vi "Check_Beam_Powers.vi"(3 "Mode":T5, 5 "Traverse line In":T2 {"Carrier_2 Q (l/min)" format="%#.2f"; "Row Duration (mins)" format="%#.1f"; "Row No" min=0; "Trace Gas Concentration (%)" min=0.0 format="%#_4f"; "Carrier_1 Q (l/min)" format="%#.4f"; "Start X" format="%#.2f"; "Start Y" format="%#.2f"; "Start Z" format="%#.2f"; "End X" format="%#.2f"; "End Y" format="%#.2f"; "End Z" format="%#.2f"; "Tunnel Speed" format="%#.2f"; "Averaging time (mins)" min=0.0 format="%#.2f"}) -> (0 "Error Message":string, 1 "Status":T1, 2 "Traverse line Out":T2 {"Carrier_2 Q (l/min)" format="%#.2f"; "Row Duration (mins)" format="%#.1f"; "Row No" min=0; "Trace Gas Concentration (%)" min=0.0 format="%#_4f"; "Carrier_1 Q (l/min)" format="%#.4f"; "Start X" format="%#.2f"; "Start Y" format="%#.2f"; "Start Z" format="%#.2f"; "End X" format="%#.2f"; "End Y" format="%#.2f"; "End Z" format="%#.2f"; "Tunnel Speed" format="%#.2f"; "Averaging time (mins)" min=0.0 format="%#.2f"})   [LabVIEW 2021]
uses:
  Gen Trav/Traverse_cluster.ctl
  Gen Trav/Spacing.ctl
  Controls/Multi_run_mode.ctl
  Controls/User_Specific_mode.ctl
  Gen Trav/Multi_Run_Status.ctl
  Gen Trav/Trav_mode.ctl
  Controls/Tunnel_Coordinates.ctl
panel:
  out "Min  Acceptable Power":dbl[](array[numeric]) format="%.3f"
  out "Initially Mirror Up?":bool
  out "Mirror Installed":string
  out "Waveform Graph":dbl[][](graph)
  out "beams to check":i32
  out "Beam Data":sgl[][](array[numeric])
  out "Light Power (mW)":dbl=8.10606551e-08 format="%#.3f"
  in  "stop":bool
  out "Powers":dbl[](array[numeric]) format="%.3f"
  out "Beam Index":i32
  # "X                      Y                   Z"
  # "X           Y          Z"
  # "Start"
  # "End"
  # "X           Y          Z"
  # "Start"
  # "End"
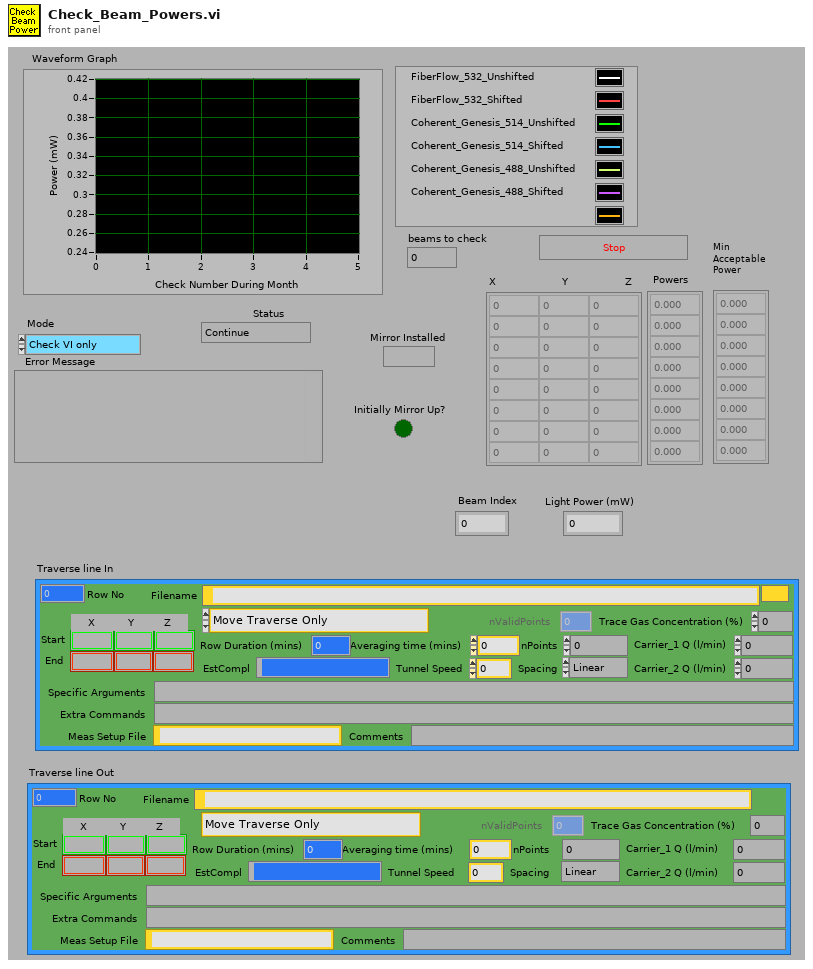
[diagram p1: front panel]
types:
  T1 = typedef "Multi_Run_Status.ctl" = enum16{"Continue", "Continue with Error", "Jump to Next Point", "Jump to Next Row", "Jump To Fall Back", "Terminate Run"}
  T2 = typedef "Traverse_cluster.ctl" = cluster{"Start X":sgl, "Start Y":sgl, "Start Z":sgl, "End X":sgl, "End Y":sgl, "End Z":sgl, "nPoints":i32, "Spacing":T3, "Filename":path, "Tunnel Speed":dbl, "Averaging time (mins)":dbl, "Extra Commands":string, "Carrier_1 Q (l/min)":dbl, "Carrier_2 Q (l/min)":dbl, "Trace Gas Concentration (%)":dbl, "Specific Arguments":string, "Comments":string, "Row No":i32, "Row Type Selector":T4, "EstCompl":string, "Row Duration (mins)":dbl, "nValidPoints":i32, "Meas Setup File":string}
  T3 = typedef "Spacing.ctl" = enum16{"Linear", "Log", "Gauss", "Specified", "N/A"}
  T4 = typedef "Multi_run_mode.ctl" = enum16{"Move Traverse Only", "Set Tunnel Speed Only", "Set Source Only", "Set Measurement Conditions", "Single Measurement", "Vertical Profile", "Lateral Profile", "Longitudinal Profile", "Multi-Axis Profile", "Explore Volume", "Auto Calibrate", "Meas Fast FID Bkgnd", "Check Beam Power", "Scanning Valve Measurement", "Run VI Named:", "Set ADAM Ch", "Wait (minutes)", "Send Message", "Synchronize With:", "Fall Back to this Row", "Turn Off Row Repeating", "Traverse 3D Volume", "Blank Row", "Jump to Fall Back Row"}
  T5 = typedef "User_Specific_mode.ctl" = enum16{"Check VI only", "Run VI"}
  T6 = cluster{"Position":dbl[], "Traverse Name":string}[][]
  T7 = typedef "Tunnel_Coordinates.ctl" = enum16{"Work in Tunnel Coordinates", "Work in Model Coordinates"}
  T8 = typedef "Trav_mode.ctl" = enum16{"Move traverse", "Read traverse position", "Teach Position"}
  T9 = cluster{"Position":dbl[], "Traverse Name":string}[]
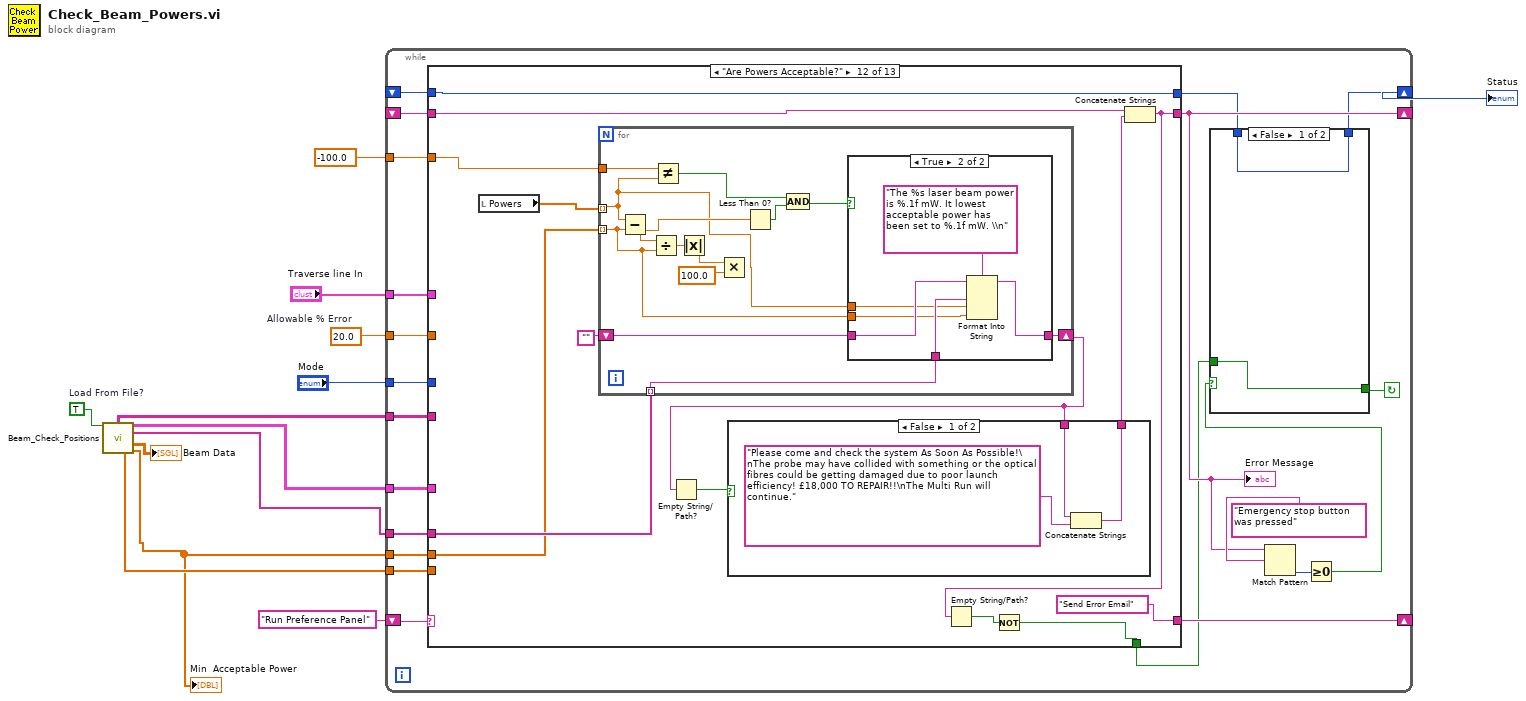
[diagram p0: block diagram]
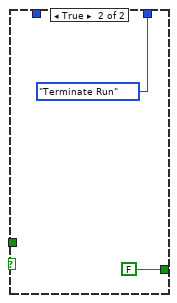
[diagram p2: hidden frame]
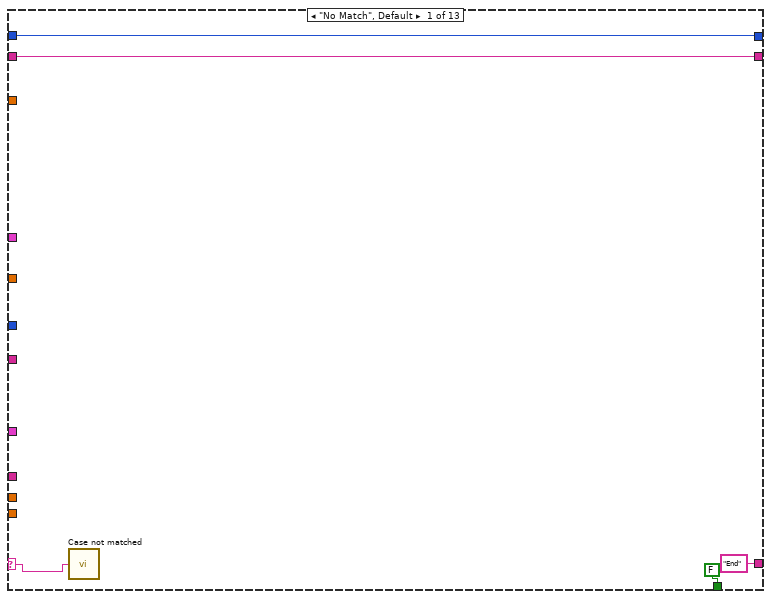
[diagram p3: hidden frame]
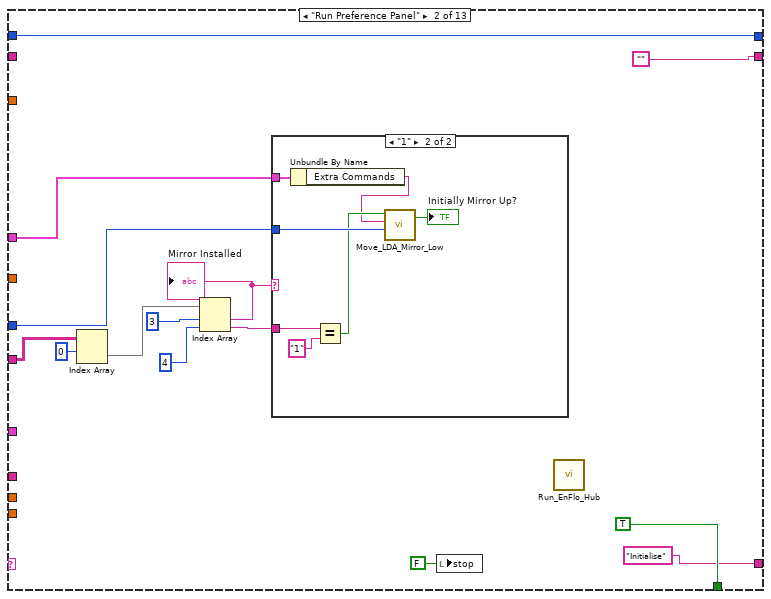
[diagram p4: hidden frame]
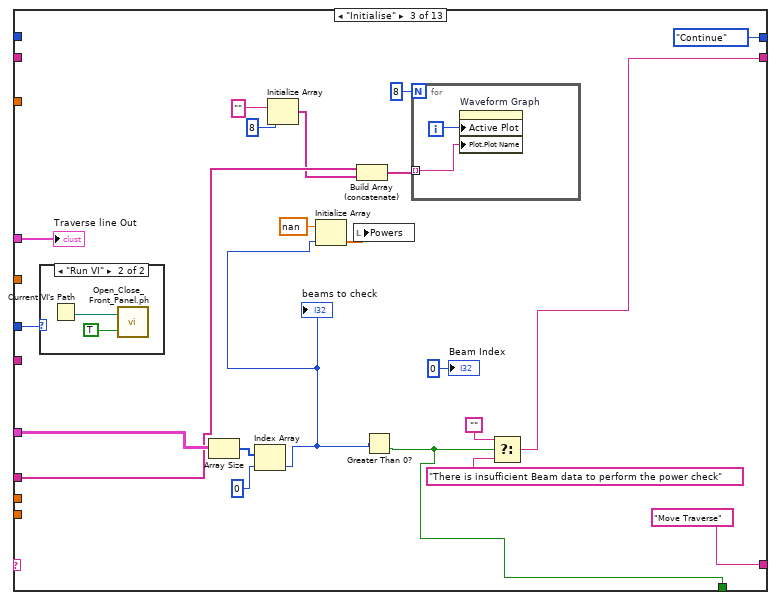
[diagram p6: hidden frame]
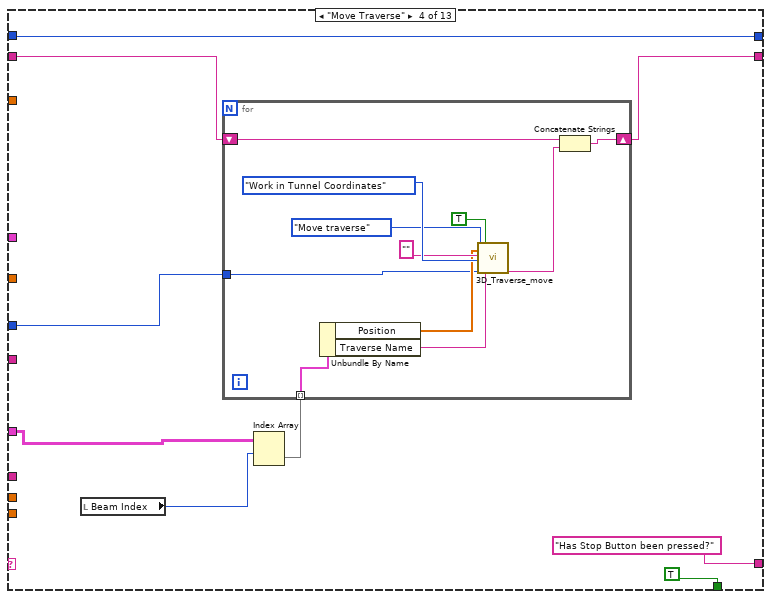
[diagram p8: hidden frame]
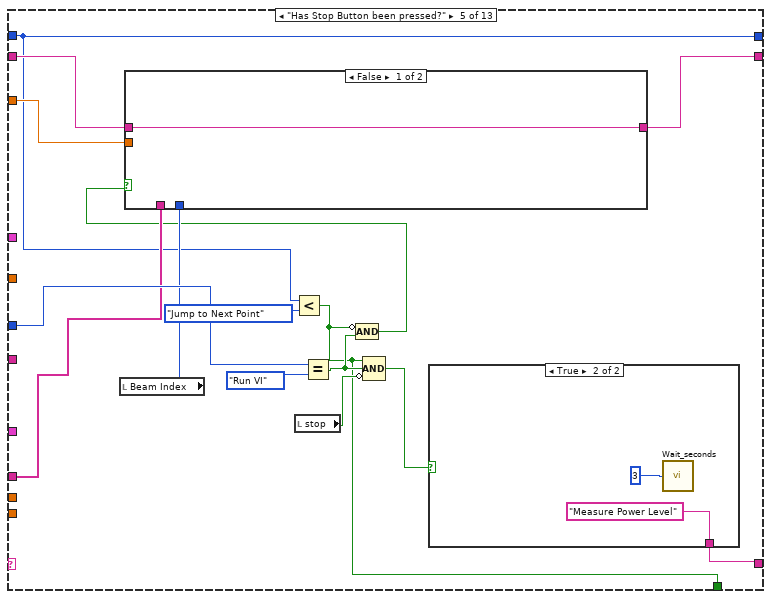
[diagram p9: hidden frame]
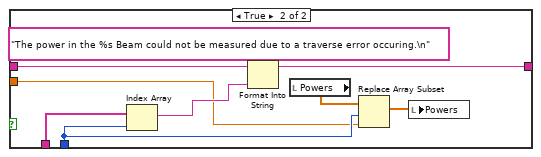
[diagram p10: hidden frame]
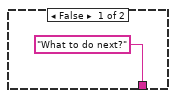
[diagram p11: hidden frame]
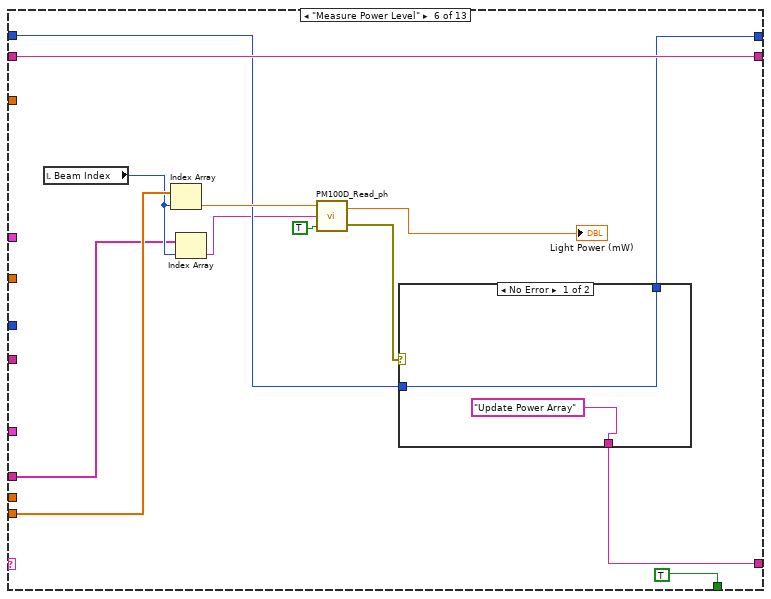
[diagram p12: hidden frame]
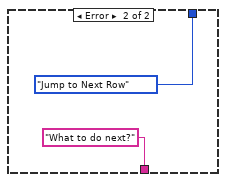
[diagram p13: hidden frame]
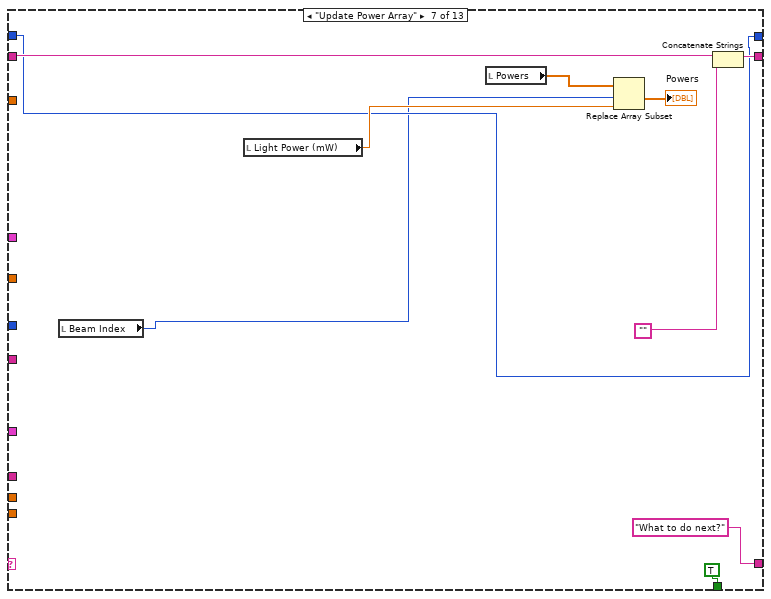
[diagram p14: hidden frame]
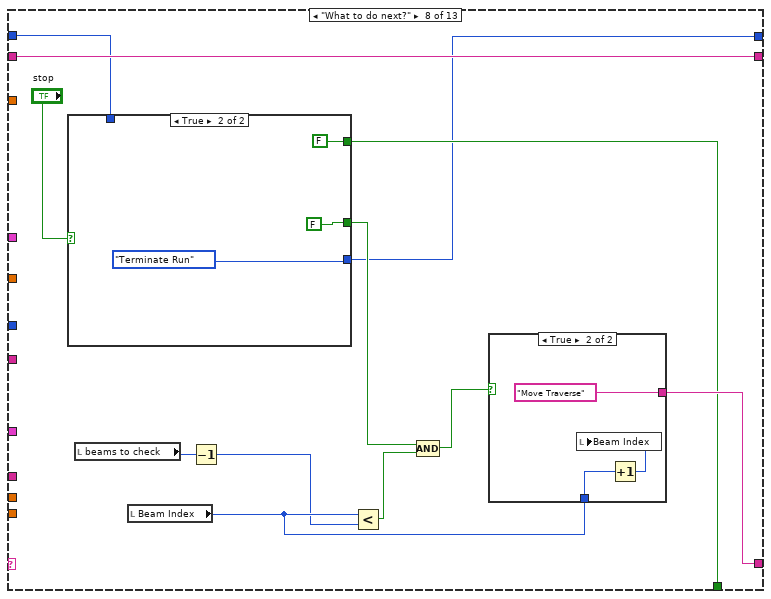
[diagram p15: hidden frame]
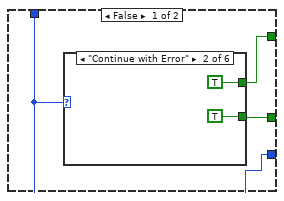
[diagram p16: hidden frame]
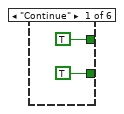
[diagram p17: hidden frame]
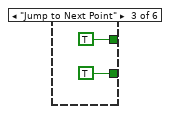
[diagram p18: hidden frame]
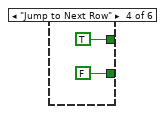
[diagram p19: hidden frame]
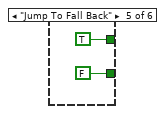
[diagram p20: hidden frame]
diagram:
  w7 = TRUE  # Load From File?
  w11 = 20.0  # Allowable % Error
  n1 = call "Beam_Check_Positions.vi"("Load From File?"=w7) -> ("More Info"=w2:string[][], "Beam Info"=w5:T6, "Beam Names"=w4:string[], "Primary Beam Positions"=→"Beam Data":dbl[][], "Wavelength (nm)"=w3:dbl[], "Power (mW)"=w1:dbl[])  [unwired: 6 in, 3 out]
  "Min  Acceptable Power" <- w1
  n2 = while {
    tunnel: -100.0 ("Element Data") -> [w27]
    tunnel: w11 -> [w29]
    shift-left: _ -> [w30]
    shift-right: [w19] -> _
    tunnel: w4 -> [w32]
    tunnel: "Traverse line In" -> [w33]
    tunnel: "Mode" -> [w34]
    shift-left: "Run Preference Panel" -> [w28]
    shift-right: [w31] -> _
    shift-right: [w15] -> w8
    shift-left: _ -> [w26]
    tunnel: w1 -> [w25]
    tunnel: w5 -> [w24]
    tunnel: w3 -> [w23]
    tunnel: w2 -> [w22]
    stop <- w17 continue-if-true
    n3 = case shown="\"Are Powers Acceptable?\"" w28 {
      selector: w28 -> [w39 _ _ _ _ _ _ _ _ _ _ _ _]
      tunnel: w33 -> [_ w44 w85 _ _ _ _ _ _ w207 _ _ _]
      tunnel: w34 -> [_ w47 w84 w90 w122 _ _ _ w203 w205 _ _ _]
      tunnel: w32 -> [_ _ w67 _ w120 w139 _ _ _ w210 _ w261 _]
      tunnel: [FALSE ("Update Datum Powers?") TRUE ("Update Datum Powers?") w78 TRUE w111 TRUE TRUE w169 w199 TRUE ("Update Datum Powers?") w229 w250 FALSE ("Update Datum Powers?")] -> w16
      tunnel: ["End" "Initialise" "Move Traverse" "Has Stop Button been pressed?" w121 w141 "What to do next?" w171 "Log Beam Power Readings" "Is Laser on Full Power?" ("f") "Are Powers Acceptable?" ("f") "Send Error Email" "End"] -> w31
      tunnel: w30 -> [w41 _ _ w94 w118 w149 w161 w173 w202 w213 w226 w259 w291]
      tunnel: [w41 "" w79 w93 w119 w149 w160 w173 w202 w213 w226 w249 ""] -> w19
      tunnel: w29 -> [_ _ _ _ _ _ _ _ _ _ _ _ _]
      tunnel: w27 -> [_ _ _ _ w117 _ _ _ _ _ _ w257 _]
      tunnel: [w40 w56 Multi_Run_Status."Continue" ("Status") w92 w110 w143 w156 w167 w201 w214 w227 w256 w287] -> w14
      tunnel: w26 -> [w40 w56 _ w92 w110 w142 w156 w168 w201 w214 w227 w256 w287]
      tunnel: w25 -> [_ _ _ _ _ _ _ _ _ _ _ w252 _]
      tunnel: w24 -> [_ _ w74 w91 _ _ _ _ _ _ _ _ _]
      tunnel: w23 -> [_ _ _ _ _ w147 _ _ _ _ _ _ _]
      tunnel: w22 -> [_ w52 _ _ _ _ _ _ _ _ w233 _ _]
      frame "No Match", Default {
        n4 = call "Case not matched.vi"("Case Name not Matched"=w39) -> ()
      }
      frame "Run Preference Panel" {
        n5 = Index Array(array=w52, index (row)=0) -> (element=w50:string[])  [unwired: 1 in]
        n6 = Index Array(array=w50, index #1=3 ("index"), index #2=4 ("index")) -> (element #1=w46:string, element #2=w45:string)
        "Mirror Installed" <- w46
        n7 = case shown="\"1\"" w46 {
          tunnel: w47 -> [_ w64]
          tunnel: w45 -> [_ w63]
          tunnel: w44 -> [_ w60]
          frame Default {
          }
          frame "1" {
            n8 = Unbundle By Name(w60) -> ("Extra Commands"=w59:string)
            n9 = Equal?(x=w63, y="1") -> (x = y?=w61:bool)
            n10 = call "Move_LDA_Mirror_Low.vi"("Mode"=w64, "Extra Commands"=w59, "Mirror Up?"=w61) -> ("Initially Mirror Up?"=→"Initially Mirror Up?":bool)  [unwired: 1 in, 1 out]
          }
        }
        n11 = local write "stop"(FALSE ("stop")) -> ()
        n12 = call "Run_EnFlo_Hub.vi"() -> ()  [unwired: 1 in, 7 out]
      }
      frame "Initialise" {
        n13 = case shown="\"Run VI\"" w84 {
          frame "Check VI only" {
          }
          frame "Run VI" {
            n14 = Current VI's Path() -> (path=w88:path)
            n15 = call "Open_Close_Front_Panel.ph.vi"("openWindow (T)"=TRUE ("Front Panel Window:Open"), "VI path"=w88) -> ()  [unwired: 2 out]
          }
        }
        n16 = Array Size(array=w74) -> (size(s)=w77:i32[])
        n17 = Index Array(array=w77, index=0) -> (element=w71:i32)
        "beams to check" <- w71
        n18 = Initialize Array("", 8 ("dimension size")) -> (w66:string[])
        n19 = Initialize Array(nan ("Numeric"), w71) -> (w73:dbl[])
        n20 = local write "Powers"(w73) -> ()
        n21 = Build Array (concatenate)(w67, w66) -> (w65:string[])
        n22 = Greater Than 0?(x=w71) -> (x > 0?=w78:bool)
        n23 = for {
          N: 8 -> [_]
          tunnel: w65 -> [w87] mode=indexing
          i -> [w86]
          n24 = property on="Waveform Graph" class="WFGraph (strict)"("Active Plot"=w86, "Plot.Plot Name"=w87) -> ()  [unwired: 2 in, 2 out]
        }
        n25 = Select(t="", s=w78, f="There is insufficient Beam data to perform the power check") -> (s? t:f=w79:string)
        "Beam Index" <- 0 ("Numeric")
        "Traverse line Out" <- w85
      }
      frame "Move Traverse" {
        n26 = local read "Beam Index"() -> (w96:i32)
        n27 = Index Array(array=w91, index (row)=w96) -> (element=w95:T9)  [unwired: 1 in]
        n28 = for {
          tunnel: w95 -> [w105] mode=indexing
          shift-right: [w102] -> w93
          shift-left: w94 -> [w101]
          tunnel: w90 -> [w99]
          n29 = Unbundle By Name(w105) -> ("Position"=w104:dbl[], "Traverse Name"=w103:string)
          n30 = call "3D_Traverse_move.vi"("Mode"=Trav_mode."Move traverse", "Position"=w104, "Extra command String"="", "Work in Tunnel Coordinates"=Tunnel_Coordinates."Work in Tunnel Coordinates", "Simulate/Run"=w99, "Route Checking?"=TRUE, "Traverse name"=w103) -> ("Error String"=w100:string)  [unwired: 9 in, 3 out]
          n31 = Concatenate Strings(w101, w100) -> (w102:string)
        }
      }
      frame "Has Stop Button been pressed?" {
        n32 = local read "Beam Index"() -> (w116:i32)
        n33 = Less?(x=w110, y=Multi_Run_Status."Jump to Next Point" ("Status")) -> (x < y?=w111:bool)
        n34 = local read "stop"() -> (w115:bool)
        n35 = Equal?(x=w122, y=User_Specific_mode."Run VI" ("Mode")) -> (x = y?=w113:bool)
        n36 = Compound Arithmetic op=AND(invert w111, w113) -> (w112:bool)
        n37 = case shown="False" w112 {
          tunnel: w116 -> [_ w127]
          tunnel: w120 -> [_ w134]
          tunnel: w118 -> [w125 w131]
          tunnel: [w125 w130] -> w119
          tunnel: w117 -> [_ w126]
          frame False {
          }
          frame True {
            n38 = Index Array(array=w134, index=w127) -> (element=w133:string)
            n39 = Format Into String(format string="The power in the %s Beam could not be measured due to a traverse error occuring.\n" ("Format String"), initial string=w131, w133) -> (resulting string=w130:string)  [unwired: 1 in, 1 out]
            n40 = local read "Powers"() -> (w129:dbl[])
            n41 = Replace Array Subset(array=w129, new element=w126, index=w127) -> (w128:dbl[])
            n42 = local write "Powers"(w128) -> ()
          }
        }
        n43 = Compound Arithmetic op=AND(w111, w113, invert w115) -> (w114:bool)
        n44 = case shown="True" w114 {
          tunnel: ["What to do next?" "Measure Power Level"] -> w121
          frame False {
          }
          frame True {
            n45 = call "Wait_seconds.vi"("Seconds to wait"=u32 3) -> ()
          }
        }
      }
      frame "Measure Power Level" {
        n46 = local read "Beam Index"() -> (w140:i32)
        n47 = Index Array(array=w147, index=w140) -> (element=w146:dbl)
        n48 = Index Array(array=w139, index=w140) -> (element=w138:string)
        n49 = call "PM100D_Read_ph.vi"("stop"=TRUE, "Beam Name"=w138, "Wavelength (0.0)"=w146) -> ("error out"=w144:errorcluster, "Average Power (mW)"=→"Light Power (mW)":dbl)
        n50 = case shown="No Error" w144 {
          tunnel: [w152 Multi_Run_Status."Jump to Next Row" ("Status")] -> w143
          tunnel: w142 -> [w152 _]
          tunnel: ["Update Power Array" "What to do next?"] -> w141
          frame No Error {
          }
          frame Error {
          }
        }
      }
      frame "Update Power Array" {
        n51 = local read "Beam Index"() -> (w155:i32)
        n52 = local read "Light Power (mW)"() -> (w157:dbl)
        n53 = local read "Powers"() -> (w163:dbl[])
        n54 = Replace Array Subset(array=w163, new element=w157, index=w155) -> (→"Powers":dbl[])
        n55 = Concatenate Strings(w161, "") -> (w160:string)
      }
      frame "What to do next?" {
        n56 = case shown="True" "stop" {
          tunnel: [w179 FALSE] -> w170
          tunnel: [w178 FALSE] -> w169
          tunnel: w168 -> [w177 _]
          tunnel: [w177 Multi_Run_Status."Terminate Run" ("Status")] -> w167
          frame False {
            n57 = case shown="\"Continue with Error\"" w177 {
              tunnel: [TRUE TRUE TRUE FALSE FALSE FALSE] -> w179
              tunnel: [TRUE TRUE TRUE TRUE TRUE FALSE] -> w178
              frame "Continue" {
              }
              frame "Continue with Error" {
              }
              frame "Jump to Next Point" {
              }
              frame "Jump to Next Row" {
              }
              frame "Jump To Fall Back" {
              }
              frame "Terminate Run" {
              }
            }
          }
          frame True {
          }
        }
        n58 = local read "beams to check"() -> (w166:i32)
        n59 = local read "Beam Index"() -> (w174:i32)
        n60 = Decrement(x=w166) -> (x-1=w165:i32)
        n61 = Less?(x=w174, y=w165) -> (x < y?=w176:bool)
        n62 = Compound Arithmetic op=AND(w170, w176) -> (w175:bool)
        n63 = case shown="True" w175 {
          tunnel: w174 -> [_ w198]
          tunnel: ["In Run Mode?" "Move Traverse"] -> w171
          frame False {
          }
          frame True {
            n64 = Increment(x=w198) -> (x+1=w197:i32)
            n65 = local write "Beam Index"(w197) -> ()
          }
        }
      }
      frame "In Run Mode?" {
        n66 = Equal?(x=w203, y=User_Specific_mode."Run VI" ("Mode")) -> (x = y?=w199:bool)
      }
      frame "Log Beam Power Readings" {
        n67 = local read "Mirror Installed"() -> (w206:string)
        n68 = local read "Powers"() -> (w211:dbl[])
        n69 = local read "Beam Data"() -> (w216:sgl[][])
        n70 = case shown="\"1\"" w206 {
          tunnel: w207 -> [_ w220]
          tunnel: w205 -> [_ w217]
          frame Default {
          }
          frame "1" {
            n71 = Unbundle By Name(w220) -> ("Extra Commands"=w219:string)
            n72 = local read "Initially Mirror Up?"() -> (w218:bool)
            n73 = call "Move_LDA_Mirror_Low.vi"("Mode"=w217, "Extra Commands"=w219, "Mirror Up?"=w218) -> ()  [unwired: 1 in, 2 out]
          }
        }
        n74 = for {
          tunnel: w216 -> [w225] mode=indexing
          tunnel: w211 -> [w222] mode=indexing
          tunnel: [w221] -> w215 mode=indexing
          n75 = Array Subset(array=w225, length=3 ("Array Length")) -> (w223:sgl[])  [unwired: 1 in]
          n76 = Build Array (concatenate)(w223, w222) -> (w221:dbl[])
        }
        n77 = call "Log_beam_power.vi"("Message"=w213, "Beam Names"=w210, "Beam Data"=w215) -> ("Power History"=→"Waveform Graph":dbl[][])  [unwired: 2 out]
      }
      frame "Is Laser on Full Power?" {
        n78 = for {
          shift-right: [w237] -> _
          shift-left: "" -> [w239]
          tunnel: w233 -> [w240] mode=indexing
          shift-right: [w235] -> w231
          shift-left: errorcluster {"status"=FALSE, "code"=0, "source"=""} ("error in (no error)") -> [w236]
          stop <- w235 stop-if-true
          n79 = Index Array(array=w240, index=1) -> (element=w237:string)
          n80 = Equal?(x=w237, y=w239) -> (x = y?=w238:bool)
          n81 = case shown="True" w238 {
            tunnel: w237 -> [w247 _]
            tunnel: [w243 w248] -> w235
            tunnel: w236 -> [w242 w248]
            frame False {
              n82 = call "Connect to Laser_Dx_client.vi"("Laser IP Number"=w247, "error in (no error)"=w242) -> ("Laser_Dx"=w246:refnum<k7>, "error out"=w245:errorcluster, "Channel"=w244:i64)
              n83 = invoke class="IBSALaser" method="ShutterOpen"(reference=w246, error in=w245, "dev"=w244) -> (error out=w243:errorcluster)  [unwired: 2 in, 4 out]
            }
            frame True {
            }
          }
        }
        n84 = Unbundle By Name(w231) -> ("status"=w230:bool)
        n85 = Not(x=w230) -> (.not. x?=w229:bool)
      }
      frame "Are Powers Acceptable?" {
        n86 = local read "Powers"() -> (w262:dbl[])
        n87 = for {
          tunnel: w262 -> [w268] mode=indexing
          tunnel: w252 -> [w267] mode=indexing
          shift-right: [w277] -> w254
          shift-left: "" -> [w279]
          tunnel: w261 -> [w278] mode=indexing
          tunnel: w257 -> [w272]
          n88 = Subtract(x=w268, y=w267) -> (x-y=w273:dbl)
          n89 = Divide(x=w273, y=w267) -> (x/y=w275:dbl)
          n90 = Not Equal?(x=w272, y=w268) -> (x != y?=w269:bool)
          n91 = Absolute Value(x=w275) -> (abs(x)=w274:dbl)
          n92 = Multiply(x=w274, y=100.0) -> ()  [unwired: 1 out]
          n93 = Less Than 0?(x=w273) -> (x < 0?=w270:bool)
          n94 = Compound Arithmetic op=AND(w269, w270) -> (w271:bool)
          n95 = case shown="True" w271 {
            tunnel: w279 -> [w280 w285]
            tunnel: w278 -> [_ w286]
            tunnel: [w280 w284] -> w277
            tunnel: w268 -> [_ w282]
            tunnel: w267 -> [_ w281]
            frame False {
            }
            frame True {
              n96 = Format Into String(format string="The %s laser beam power is %.1f mW. It lowest acceptable power has been set to %.1f mW. \\n" ("Format String"), initial string=w285, w286, w282, w281) -> (resulting string=w284:string)  [unwired: 1 in, 1 out]
            }
          }
        }
        n97 = Empty String/Path?(string/path=w254) -> (empty?=w255:bool)
        n98 = case shown="False" w255 {
          tunnel: w254 -> [w264 w266]
          tunnel: [w263 w266] -> w253
          frame False {
            n99 = Concatenate Strings(w264, "Please come and check the system As Soon As Possible!\nThe probe may have collided with something or the optical fibres could be getting damaged due to poor launch efficiency! £18,000 TO REPAIR!!\nThe Multi Run will continue." ("Substring")) -> (w263:string)
          }
          frame True {
          }
        }
        n100 = Concatenate Strings(w259, w253) -> (w249:string)
        n101 = Empty String/Path?(string/path=w249) -> (empty?=w251:bool)
        n102 = Not(x=w251) -> (.not. x?=w250:bool)
      }
      frame "Send Error Email" {
        w295 = FALSE  # Dialog Box (T)
        n103 = Bundle By Name(cluster=errorcluster {"status"=FALSE, "code"=0, "source"=""} ("error in (no error)"), "source"=w291, "status"=TRUE ("Bundle Element")) -> (w293:errorcluster)
        n104 = call "EnFlo_Error_Handler.vi"("error in (no error)"=w293, "Error Type"="Beam Power", "Dialog Box (F)"=w295) -> ()  [unwired: 3 out]
      }
    }
    "Error Message" <- w19
    n105 = Match Pattern(string=w19, regular expression="Emergency stop button was pressed") -> (offset past match=w21:i32)  [unwired: 4 out]
    n106 = Greater Or Equal To 0?(x=w21) -> (x >= 0?=w18:bool)
    n107 = case shown="False" w18 {
      tunnel: [w36 FALSE ("t")] -> w17
      tunnel: w16 -> [w36 _]
      tunnel: [w35 Multi_Run_Status."Terminate Run" ("Status")] -> w15
      tunnel: w14 -> [w35 _]
      frame False {
      }
      frame True {
      }
    }
  }
  "Status" <- w8
